vi "Init UI.vi"(8 "error in (no error)":errorcluster, 11 "GlobalData":T2) -> (0 "error out":errorcluster)   [LabVIEW 2024]
doc: "This UI inlilize units of the system"
uses:
  controls/GlobalData.ctl
  controls/Units.ctl
  <userlib>/_OpenG.lib/lvdata/lvdata.llb/openg_variant.lvlib
panel:
  in  "Units Settings":T1={"Pressure"=enum."Pa", "Temperature"=enum."F", "Salinity"=enum."ppt", "Weight"=enum."ib"}
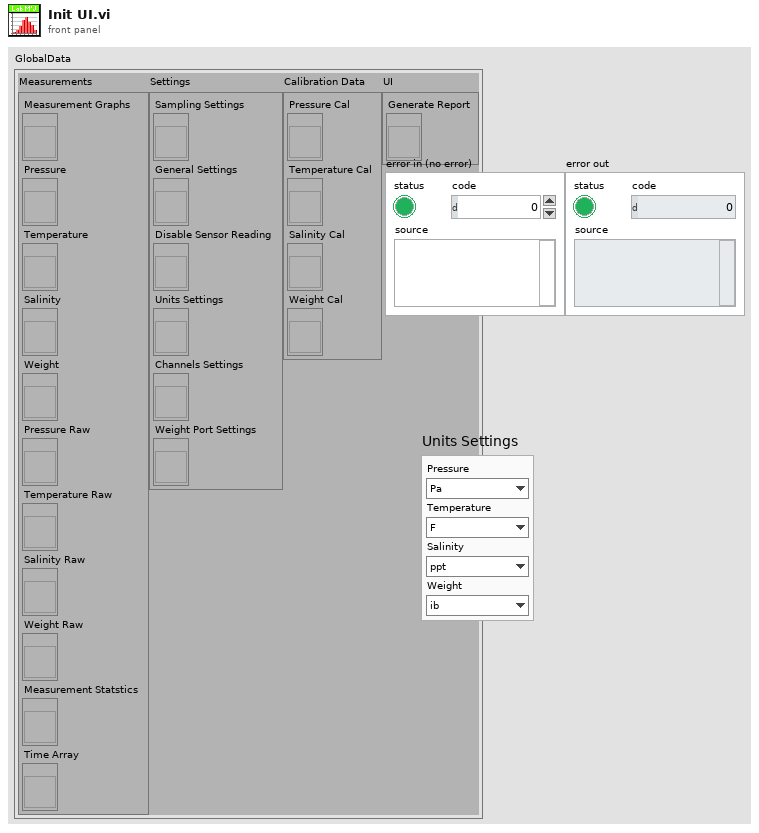
[diagram p1: front panel]
types:
  T1 = typedef "Units.ctl" = cluster{"Pressure":enum16{"PSI", "Bar", "atm", "Pa"}, "Temperature":enum16{"C", "K", "F"}, "Salinity":enum16{"ppm", "ppt", "PSU"}, "Weight":enum16{"Kg", "g", "oz", "ib"}}
  T2 = typedef "GlobalData.ctl" = cluster{"Measurements":cluster{"Measurement Graphs":refnum<vi>, "Pressure":refnum<vi>, "Temperature":refnum<vi>, "Salinity":refnum<vi>, "Weight":refnum<vi>, "Pressure Raw":refnum<vi>, "Temperature Raw":refnum<vi>, "Salinity Raw":refnum<vi>, "Weight Raw":refnum<vi>, "Measurement Statstics":refnum<vi>, "Time Array":refnum<vi>}, "Settings":cluster{"Sampling Settings":refnum<vi>, "General Settings":refnum<vi>, "Disable Sensor Reading":refnum<vi>, "Units Settings":refnum<vi>, "Channels Settings":refnum<vi>, "Weight Port Settings":refnum<vi>}, "Calibration Data":cluster{"Pressure Cal":refnum<vi>, "Temperature Cal":refnum<vi>, "Salinity Cal":refnum<vi>, "Weight Cal":refnum<vi>}, "UI":cluster{"Generate Report":refnum<vi>}}
  T3 = cluster{"Measurement Statstics":bool, "Logging Type":enum16{"Disable Log", "TDMS", "CSV"}}
  T4 = cluster{"Reading Time (ms)":u64, "Graph Time ":u16}
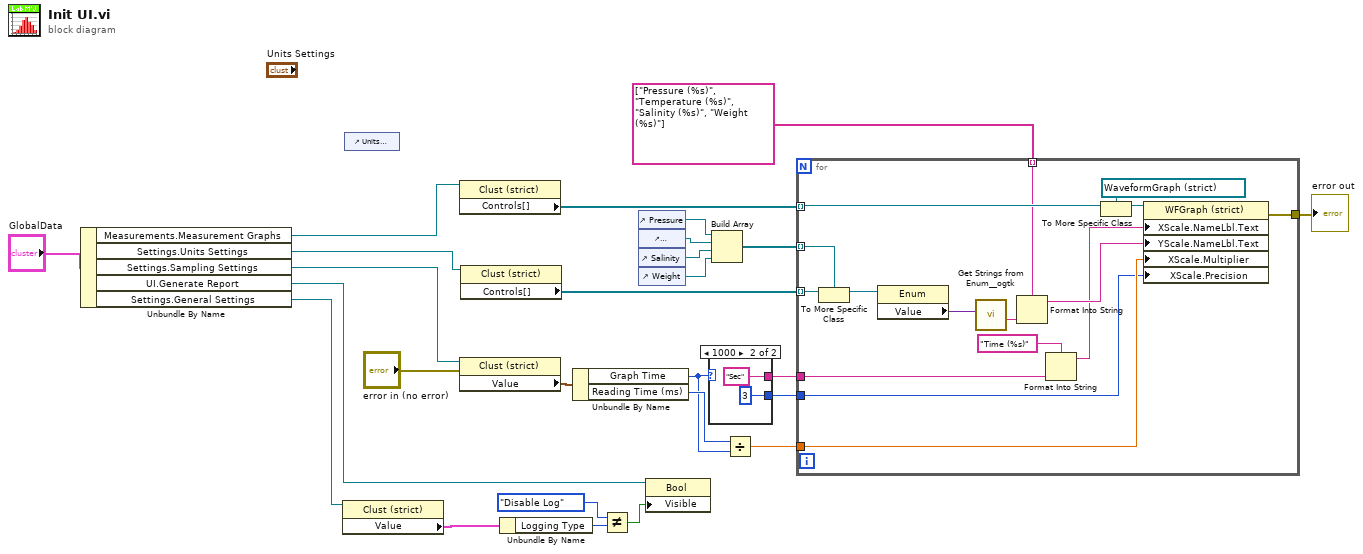
[diagram p0: block diagram]
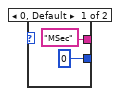
[diagram p2: hidden frame]
diagram:
  n1 = Unbundle By Name("GlobalData") -> ("Measurements.Measurement Graphs"=w24:refnum<vi>, "Settings.Units Settings"=w13:refnum<vi>, "Settings.Sampling Settings"=w20:refnum<vi>, "UI.Generate Report"=w6:refnum<vi>, "Settings.General Settings"=w5:refnum<vi>)
  n2 = property on="Property Node" class="Clust (strict)"(reference=w5) -> ("Value"=w4:T3)  [unwired: 1 in, 2 out]
  n3 = control-ref of="Units Settings"() -> ()  [unwired: 1 out]
  n4 = property on="Property Node" class="Clust (strict)"(reference=w24) -> ("Controls[]"=w23:refnum<vi>[])  [unwired: 1 in, 2 out]
  n5 = property on="Property Node" class="Clust (strict)"(reference=w20, error in="error in (no error)") -> ("Value"=w21:T4)  [unwired: 2 out]
  n6 = property on="Property Node" class="Clust (strict)"(reference=w13) -> ("Controls[]"=w22:refnum<vi>[])  [unwired: 1 in, 2 out]
  n7 = Unbundle By Name(w4) -> ("Logging Type"=w3:enum16{"Disable Log", "TDMS", "CSV"})
  n8 = Unbundle By Name(w21) -> ("Graph Time"=w18:u16, "Reading Time (ms)"=w25:u64)
  n9 = Not Equal?(x=enum16{"Disable Log", "TDMS", "CSV"}."Disable Log", y=w3) -> (x != y?=w1:bool)
  n10 = control-ref of="Pressure"() -> (w9:refnum<vi>)
  n11 = control-ref of="Temperature"() -> (w10:refnum<vi>)
  n12 = control-ref of="Salinity"() -> (w11:refnum<vi>)
  n13 = control-ref of="Weight"() -> (w12:refnum<vi>)
  n14 = property on="Property Node" class="Bool"(reference=w6, "Visible"=w1) -> ()  [unwired: 1 in, 2 out]
  n15 = case shown="1000" w18 {
    tunnel: [u64 0 ("Reading Time (ms)") u64 3 ("Reading Time (ms)")] -> w16
    tunnel: ["MSec" ("X Scale.Name Label.Text") "Sec" ("X Scale.Name Label.Text")] -> w19
    frame 0, Default {
    }
    frame 1000 {
    }
  }
  n16 = Build Array(w9, w10, w11, w12) -> (w8:refnum<vi>[])
  n17 = Divide(x=w25, y=w18) -> (x/y=w17:dbl)
  n18 = for {
    tunnel: w23 -> [w46] mode=indexing
    tunnel: w22 -> [w44] mode=indexing
    tunnel: w19 -> [w40]
    tunnel: w17 -> [w33]
    tunnel: w16 -> [w32]
    tunnel: [w38] -> w14
    tunnel: w8 -> [w34] mode=indexing
    tunnel: string[] ["Pressure (%s)", "Temperature (%s)", "Salinity (%s)", "Weight (%s)"] -> [w35] mode=indexing
    n19 = To More Specific Class(target class=w34, reference=w44) -> (specific class reference=w43:refnum<vi>)  [unwired: 1 in, 1 out]
    n20 = property on="Property Node" class="Enum"(reference=w43) -> ("Value"=w42:variant)  [unwired: 1 in, 2 out]
    n21 = call <userlib>:"Get Strings from Enum__ogtk.vi"("Enum"=w42) -> ("String Value"=w41:string)  [unwired: 7 in, 3 out]
    n22 = Format Into String(format string=w35, w41) -> (resulting string=w39:string)  [unwired: 2 in, 1 out]
    n23 = Format Into String(format string="Time (%s)", w40) -> (resulting string=w31:string)  [unwired: 2 in, 1 out]
    n24 = To More Specific Class(target class=refnum<vi> refnum ("Pressure"), reference=w46) -> (specific class reference=w36:refnum<vi>)  [unwired: 1 in, 1 out]
    n25 = property on="Property Node" class="WFGraph (strict)"(reference=w36, "XScale.NameLbl.Text"=w31, "YScale.NameLbl.Text"=w39, "XScale.Multiplier"=w33, "XScale.Precision"=w32) -> (error out=w38:errorcluster)  [unwired: 1 in, 1 out]
  }
  "error out" <- w14
